vi "Teleop.vi"(10 "Match Info":T1={"Autonomous Elapsed Seconds"=0.0, "TeleOp Elapsed Seconds"=0.0, "Disabled Elapsed Seconds"=0.0, "Visited Autonomous"=FALSE, "Visited TeleOp"=FALSE, "Visited Disabled"=FALSE, "Autonomous Settings"={"Autonomous Style"=enum."Independent", "VI Refnum"=refnum}}, 11 "Call Context":T2) -> ()   [LabVIEW 2014]
doc: "This VI is called for each TeleOp packet received from the DS where the robot is not disabled. It is often used to read from the joysticks and update I/O or to update setpoints for timed control loops. It should complete and return within 20 milliseconds or it may miss DS packets."
uses:
  <vilib>/Rock Robotics/WPI/DriverStation/WPI_DriverStationDerivedRobotMode.ctl
  <vilib>/Rock Robotics/WPI/DriverStation/WPI_DriverStationMatch Info.ctl
  <vilib>/Rock Robotics/WPI/Joystick/WPI_JoystickGetSetRefNum.vi
  <vilib>/Rock Robotics/Network Tables/SD Write Boolean Array.vi
  <vilib>/Rock Robotics/Network Tables/SD Write Numeric Array.vi
  <vilib>/Rock Robotics/Network Tables/SD Read Boolean.vi
  <vilib>/Rock Robotics/Network Tables/SD Read Number.vi
panel:
  out "Sample Slider 0":dbl(slide) scale=0.0..5.0
  out "Sample Boolean 1":bool
  out "Sample Boolean 0":bool
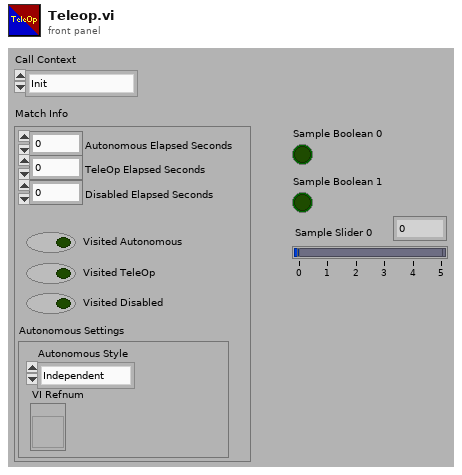
[diagram p1: front panel]
types:
  T1 = typedef "WPI_DriverStationMatch Info.ctl" = cluster{"Autonomous Elapsed Seconds":dbl, "TeleOp Elapsed Seconds":dbl, "Disabled Elapsed Seconds":dbl, "Visited Autonomous":bool, "Visited TeleOp":bool, "Visited Disabled":bool, "Autonomous Settings":cluster{"Autonomous Style":enum16{"Iterative", "Independent"}, "VI Refnum":refnum<vi>}}
  T2 = typedef "WPI_DriverStationDerivedRobotMode.ctl" = enum16{"Init", "Execute", "Stop"}
  T3 = cluster{"proportional gain (Kc)":dbl, "integral time (Ti, min)":dbl, "derivative time (Td, min)":dbl}
  T4 = typedef "WPI_JoystickDevRef.ctl" = cluster{"Device":T5}
  T5 = typedef "WPI_JoystickDeviceEnum.ctl" = enum16{"USB 0", "USB 1", "USB 2", "USB 3", "USB 4", "USB 5"}
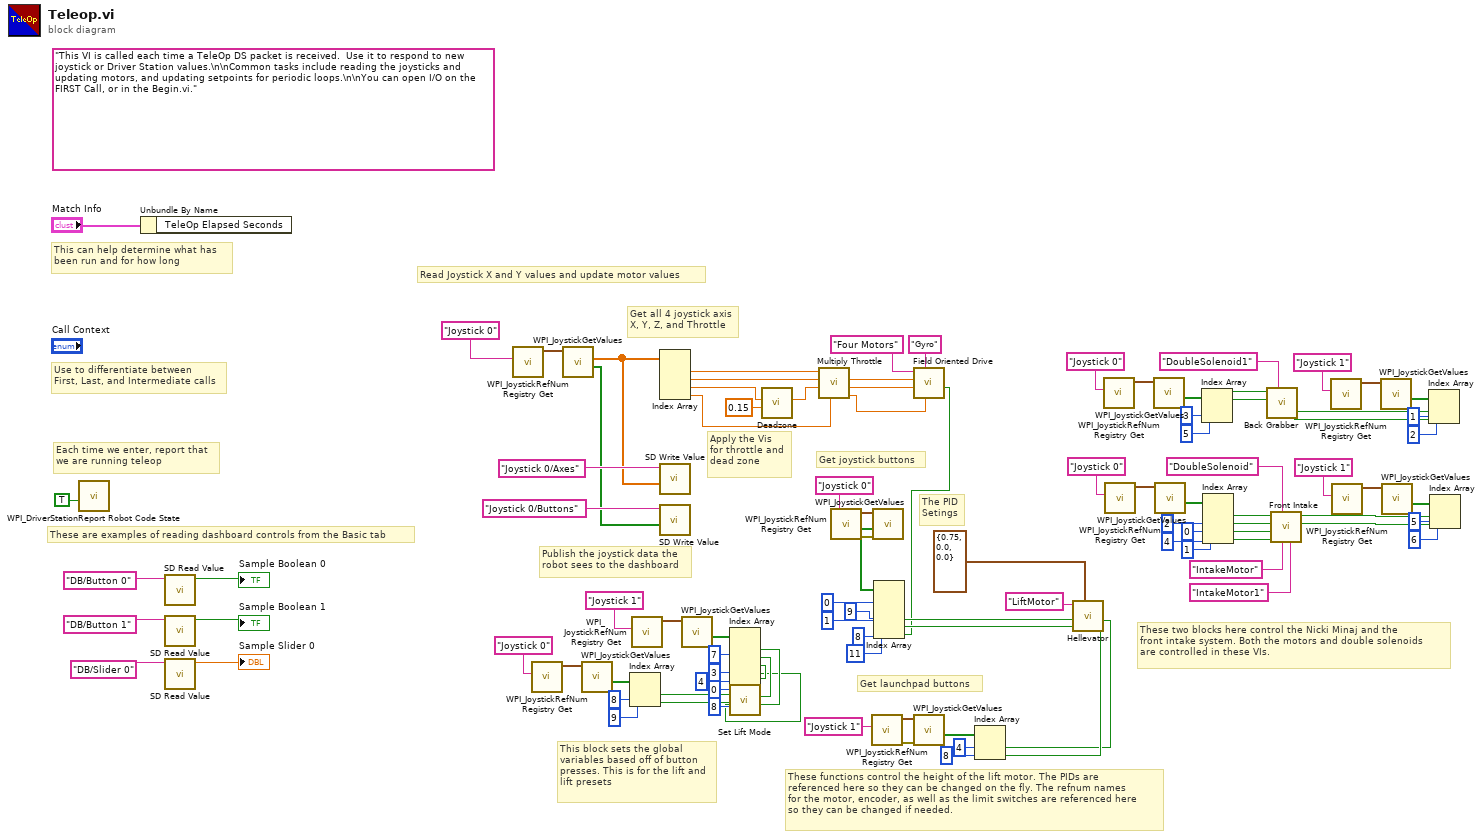
[diagram p0: block diagram]
diagram:
  (unwired) "This VI is called each time a TeleOp DS packet is received.  Use it to respond to new joystick or Driver Station values.\n\nCommon tasks include reading the joysticks and updating motors, and updating setpoints for periodic loops.\n\nYou can open I/O on the FIRST Call, or in the Begin.vi."
  # "Apply the Vis\nfor throttle and\ndead zone"
  # "These functions control the height of the lift motor. The PIDs are\nreferenced here so they can be changed on the fly. The refnum names\nfor the motor, encoder, as well as the limit switches are referenced here\nso they can be changed if needed."
  # "These two blocks here control the Nicki Minaj and the \nfront intake system. Both the motors and double solenoids\nare controlled in these VIs."
  # "This block sets the global\nvariables based off of button\npresses. This is for the lift and\nlift presets"
  # "Get launchpad buttons"
  # "The PID\nSetings"
  # "Get joystick buttons"
  # "Get all 4 joystick axis\nX, Y, Z, and Throttle"
  # "These are examples of reading dashboard controls from the Basic tab"
  # "Publish the joystick data the\nrobot sees to the dashboard"
  # "Each time we enter, report that\nwe are running teleop"
  # "Use to differentiate between\nFirst, Last, and Intermediate calls"
  # "This can help determine what has\nbeen run and for how long"
  # "Read Joystick X and Y values and update motor values"
  n1 = call <vilib>:"WPI_DriverStationReport Robot Code State.vi"("TeleOp"=TRUE ("Autonomous")) -> ()  [unwired: 10 in, 1 out]
  n2 = Unbundle By Name("Match Info") -> ()  [unwired: 1 out]
  n3 = call-poly <vilib>:"SD Read Value.vi"("Name"="DB/Button 0" ("refnum name")) -> ("Boolean"=→"Sample Boolean 0":bool)  [unwired: 8 in, 2 out]
  n4 = call-poly <vilib>:"SD Read Value.vi"("Name"="DB/Button 1" ("refnum name")) -> ("Boolean"=→"Sample Boolean 1":bool)  [unwired: 8 in, 2 out]
  n5 = call-poly <vilib>:"SD Read Value.vi"("Name"="DB/Slider 0" ("refnum name")) -> ("Numeric"=→"Sample Slider 0":dbl)  [unwired: 8 in, 2 out]
  n6 = call <vilib>:"WPI_JoystickRefNum Registry Get.vi"("refnum name"="Joystick 0") -> ("JoystickDevRef"=w101:T4)  [unwired: 1 in, 9 out]
  n7 = call <vilib>:"WPI_JoystickRefNum Registry Get.vi"("refnum name"="Joystick 0") -> ("JoystickDevRef"=w62:T4)  [unwired: 1 in, 9 out]
  n8 = call <vilib>:"WPI_JoystickGetValues.vi"("JoystickDevRef"=w101) -> ("Buttons"=w76:bool[], "Axes"=w91:dbl[])  [unwired: 6 in, 3 out]
  n9 = call <vilib>:"WPI_JoystickGetValues.vi"("JoystickDevRef"=w62) -> ("Buttons"=w51:bool[])  [unwired: 6 in, 4 out]
  n10 = Index Array(array=w51, index #1=8 ("index"), index #2=9 ("index")) -> (element #1=w52:bool, element #2=w61:bool)
  n11 = call <vilib>:"WPI_JoystickRefNum Registry Get.vi"("refnum name"="Joystick 1") -> ("JoystickDevRef"=w59:T4)  [unwired: 1 in, 9 out]
  n12 = Index Array(array=w91) -> (element #1=w65:dbl, element #2=w66:dbl, element #3=w75:dbl, element #4=w64:dbl)  [unwired: 4 in]
  n13 = call-poly <vilib>:"SD Write Value.vi"("Numeric Array"=w91, "Name"="Joystick 0/Axes") -> ()  [unwired: 8 in, 2 out]
  n14 = call-poly <vilib>:"SD Write Value.vi"("Boolean Array"=w76, "Name"="Joystick 0/Buttons") -> ()  [unwired: 8 in, 2 out]
  n15 = call <vilib>:"WPI_JoystickGetValues.vi"("JoystickDevRef"=w59) -> ("Buttons"=w58:bool[])  [unwired: 6 in, 4 out]
  n16 = Index Array(array=w58, index #1=7 ("index"), index #2=3 ("index"), index #3=0 ("index"), index #4=8 ("index"), index #5=4 ("index")) -> (element #1=w41:bool, element #2=w42:bool, element #3=w43:bool, element #4=w39:bool, element #5=w37:bool)
  n17 = call "Set Lift Mode.vi"("PresetLow"=w41, "PresetMid"=w42, "PresetHigh"=w43, "LP Down"=w37, "LP Up"=w39, "Joy Down"=w61, "Joy Up"=w52) -> ()  [unwired: 5 in]
  n18 = call "Deadzone.vi"("Deadzone"=0.15, "Joystick Input"=w75) -> ("Joystick Output"=w67:dbl)  [unwired: 9 in]
  n19 = call "Multiply Throttle.vi"("Joystick Throttle Input"=w64, "Joystick Z Input"=w67, "Joystick Y Input"=w66, "Joystick X Input"=w65) -> ("Joystick Z Output"=w48:dbl, "Joystick Y Output"=w49:dbl, "Joystick X Output"=w50:dbl)  [unwired: 5 in]
  n20 = call <vilib>:"WPI_JoystickRefNum Registry Get.vi"("refnum name"="Joystick 0") -> ("error out"=w90:errorcluster, "JoystickDevRef"=w89:T4)  [unwired: 9 in]
  n21 = call <vilib>:"WPI_JoystickRefNum Registry Get.vi"("refnum name"="Joystick 1") -> ("error out"=w82:errorcluster, "JoystickDevRef"=w81:T4)  [unwired: 9 in]
  n22 = call <vilib>:"WPI_JoystickGetValues.vi"("error in (no error)"=w90, "JoystickDevRef"=w89) -> ("Buttons"=w87:bool[])  [unwired: 5 in, 4 out]
  n23 = Index Array(array=w87, index #1=0 ("index"), index #2=1 ("index"), index #3=9 ("index"), index #4=8 ("index"), index #5=11 ("index")) -> (element #3=w72:bool, element #4=w68:bool, element #5=w44:bool)  [unwired: 2 out]
  n24 = call "Field Oriented Drive.vi"("FIeld Oriented Drive Toggle Button"=w44, "Joystick Z Output"=w48, "Gyro Refnum Name"="Gyro", "Joystick Y Output"=w49, "Joystick X Output"=w50, "Motor Refnum Name"="Four Motors") -> ()  [unwired: 6 in]
  n25 = call <vilib>:"WPI_JoystickGetValues.vi"("error in (no error)"=w82, "JoystickDevRef"=w81) -> ("Buttons"=w79:bool[])  [unwired: 5 in, 4 out]
  n26 = Index Array(array=w79, index #1=4 ("index"), index #2=8 ("index")) -> (element #1=w70:bool, element #2=w71:bool)
  n27 = call "Hellevator.vi"("Lift Launchpad 2"=w71, "Lift Launchpad 1"=w70, "PID gains"=T3 {"proportional gain (Kc)"=0.75, "integral time (Ti, min)"=0.0, "derivative time (Td, min)"=0.0}, "Lift Button 2"=w68, "Lift Button 1"=w72, "Motor Refnum Name"="LiftMotor") -> ()  [unwired: 6 in]
  n28 = call <vilib>:"WPI_JoystickRefNum Registry Get.vi"("refnum name"="Joystick 0") -> ("JoystickDevRef"=w34:T4)  [unwired: 1 in, 9 out]
  n29 = call <vilib>:"WPI_JoystickRefNum Registry Get.vi"("refnum name"="Joystick 0") -> ("JoystickDevRef"=w20:T4)  [unwired: 1 in, 9 out]
  n30 = call <vilib>:"WPI_JoystickGetValues.vi"("JoystickDevRef"=w34) -> ("Buttons"=w31:bool[])  [unwired: 6 in, 4 out]
  n31 = call <vilib>:"WPI_JoystickGetValues.vi"("JoystickDevRef"=w20) -> ("Buttons"=w17:bool[])  [unwired: 6 in, 4 out]
  n32 = Index Array(array=w31, index #1=3 ("index"), index #2=5 ("index")) -> (element #1=w30:bool, element #2=w29:bool)
  n33 = Index Array(array=w17, index #1=2 ("index"), index #2=4 ("index"), index #3=0 ("index"), index #4=1 ("index")) -> (element #1=w10:bool, element #2=w9:bool, element #3=w6:bool, element #4=w5:bool)
  n34 = call <vilib>:"WPI_JoystickRefNum Registry Get.vi"("refnum name"="Joystick 1") -> ("JoystickDevRef"=w27:T4)  [unwired: 1 in, 9 out]
  n35 = call <vilib>:"WPI_JoystickRefNum Registry Get.vi"("refnum name"="Joystick 1") -> ("JoystickDevRef"=w15:T4)  [unwired: 1 in, 9 out]
  n36 = call <vilib>:"WPI_JoystickGetValues.vi"("JoystickDevRef"=w27) -> ("Buttons"=w24:bool[])  [unwired: 6 in, 4 out]
  n37 = call <vilib>:"WPI_JoystickGetValues.vi"("JoystickDevRef"=w15) -> ("Buttons"=w12:bool[])  [unwired: 6 in, 4 out]
  n38 = Index Array(array=w24, index #1=1 ("index"), index #2=2 ("index")) -> (element #1=w23:bool, element #2=w22:bool)
  n39 = call "Back Grabber.vi"("Launchpad Button 2"=w22, "Launchpad Button 1"=w23, "Solenoid Refnum Name"="DoubleSolenoid1", "Joystick Button 2"=w29, "Joystick Button 1"=w30) -> ()  [unwired: 7 in]
  n40 = Index Array(array=w12, index #1=5 ("index"), index #2=6 ("index")) -> (element #1=w8:bool, element #2=w7:bool)
  n41 = call "Front Intake.vi"("Launchpad Button Backward"=w7, "Launchpad Button Forward"=w8, "Intake Motor 2 Refnum Name"="IntakeMotor1", "Intake Motor 1 Refnum Name"="IntakeMotor", "Solenoid Refnum Name"="DoubleSolenoid", "Joystick Button Spin"=w5, "Joystick Button In"=w6, "Joystick Button Backward"=w9, "Joystick Button Forward"=w10) -> ()  [unwired: 3 in]
